vi "Segregate parameters.vi"(10 "Input statement":string, 11 "Number of parameters":i32) -> (2 "Parameter values array":string[](array[string]))   [LabVIEW 2019, in "ZenGage v3.0 UI.lvclass"]
uses:
  ZenGage v3.0 UI.lvclass
  <vilib>/regexp/Match Regular Expression.xnode
panel:
  # "e"
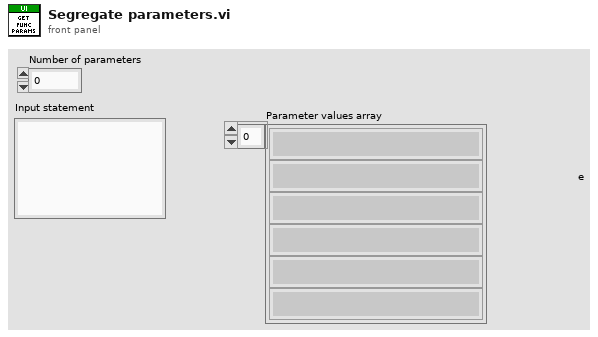
[diagram p1: front panel]
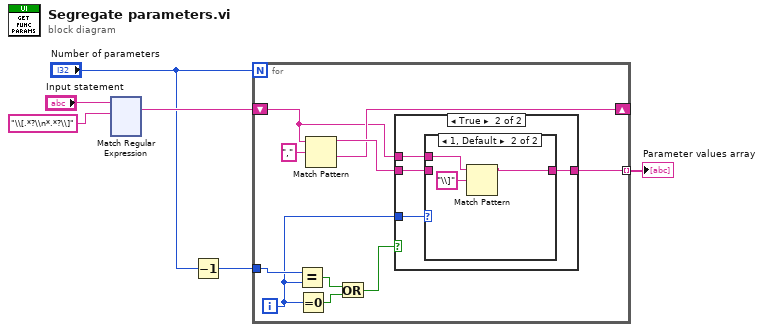
[diagram p0: block diagram]
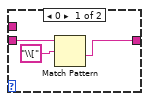
[diagram p3: hidden frame]
diagram:
  n1 = xnode "Match Regular Expression"("input string"="Input statement", "regular expression"="\\[.*?\\n*.*?\\]") -> ("whole match"=w4:string)  [unwired: 4 in, 4 out]
  n2 = Decrement(x="Number of parameters") -> (x-1=w2:i32)
  n3 = for {
    N: "Number of parameters" -> [_]
    tunnel: w2 -> [w16]
    tunnel: [w10] -> w1 mode=indexing
    shift-right: [w9] -> _
    shift-left: w4 -> [w7]
    i -> [w8]
    n4 = Equal?(x=w16, y=w8) -> (x = y?=w15:bool)
    n5 = Equal To 0?(x=w8) -> (x = 0?=w14:bool)
    n6 = Match Pattern(string=w7, regular expression=",") -> (before substring=w11:string, after substring=w9:string)  [unwired: 1 in, 2 out]
    n7 = Or(x=w15, y=w14) -> (x .or. y?=w13:bool)
    n8 = case shown="True" w13 {
      tunnel: w11 -> [w17 w20]
      tunnel: [w17 w19] -> w10
      tunnel: w8 -> [_ w21]
      tunnel: w7 -> [_ w18]
      frame False {
      }
      frame True {
        n9 = case shown="1, Default" w21 {
          tunnel: w20 -> [w24 _]
          tunnel: [w22 w25] -> w19
          tunnel: w18 -> [_ w26]
          frame 0 {
            n10 = Match Pattern(string=w24, regular expression="\\[") -> (after substring=w22:string)  [unwired: 1 in, 3 out]
          }
          frame 1, Default {
            n11 = Match Pattern(string=w26, regular expression="\\]") -> (before substring=w25:string)  [unwired: 1 in, 3 out]
          }
        }
      }
    }
  }
  "Parameter values array" <- w1
